vi "FTW-Actor-LaunchChildActor-Path.vi"(0 "FTW-ActorInstance In":refnum<class "FTW-ActorInstance.lvclass">, 5 "Configuration":string="{\n  \"Identity\": \"ActorName\",\n  \"DebugEnableInboxLogging\": false,\n  \"DebugEnableJobLogging\": false,\n  \"InboxAddress\": \"inproc://*\",\n  \"DebugShowPanel\": false\n}", 7 "Actor VI Path":path, 9 "Timeout":i32=-2 format="%dmsec", 11 "error in":errorcluster) -> (4 "FTW-ActorInstance Out":refnum<class "FTW-ActorInstance.lvclass">, 6 "Initialized Response":string, 8 "Instance Inbox Address":string, 10 "Identity":string, 15 "error out":errorcluster)   [LabVIEW 2018, in "FTW-ActorInstance.lvclass"]
doc: "This is the spawn new actor that was used for a while. It lacks the minimum strict inputs required to launch an actor."
uses:
  FTW-ActorInstance.lvclass
  Connector/FTW-ActorConnector.lvclass
  4a73fd1e-9fc2-4821-946b-9eb06f56bf7f.vi
  JSON/core/FTW-JSON-Core-EncodingFlags.vi
  Reflection/FTW-Reflection-Type.vi
  JSON/FTW-JSON-Parse.vi
  container/FTW-Container-GetFlattenedValue.vi
panel:
  # "Inputs"
  # "Outputs"
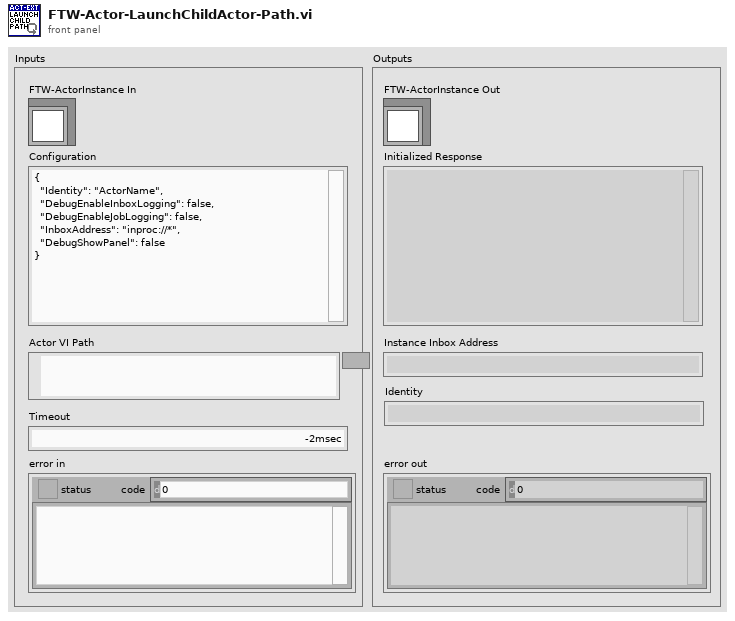
[diagram p1: front panel]
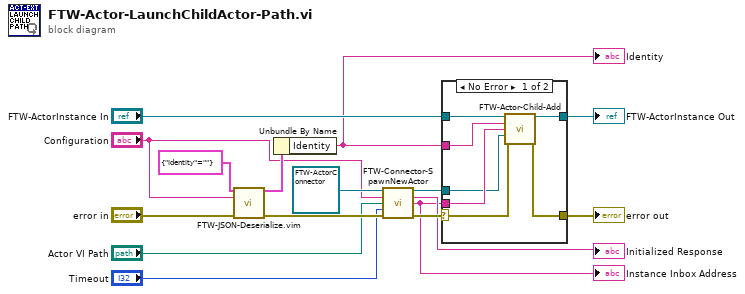
[diagram p0: block diagram]
diagram:
  n1 = call "FTW-JSON-Deserialize.vim"("Type In"=cluster{"Identity":string} {"Identity"=""}, "JSON String"="Configuration", "error in"="error in") -> ("Type Out"=w15:cluster{"Identity":string}, "error out"=w13:errorcluster)  [unwired: 11 in]
  n2 = Unbundle By Name(w15) -> ("Identity"=w2:string)
  "Identity" <- w2
  n3 = call "FTW-Connector-SpawnNewActor.vi"("FTW Actor Connector Type"=refnum<class "FTW-ActorConnector.lvclass"> refnum, "Configuration"="Configuration", "Actor VI Filepath"="Actor VI Path", "Timeout"="Timeout", "error in"=w13) -> ("FTW Actor Connector"=w11:refnum<class "FTW-ActorConnector.lvclass">, "Initialized Response"=→"Initialized Response":string, "Instance Inbox Address"=w5:string, "error out"=w12:errorcluster)  [unwired: 7 in]
  "Instance Inbox Address" <- w5
  n4 = case shown="No Error" w12 {
    selector: w12 -> [w23 w24]
    tunnel: "FTW-ActorInstance In" -> [w21 w25]
    tunnel: [w20 w25] -> w7
    tunnel: [w22 w24] -> w4
    tunnel: w2 -> [w19 _]
    tunnel: w5 -> [w18 _]
    tunnel: w11 -> [w17 _]
    frame No Error {
      n5 = call "FTW-Actor-Child-Add.vi"("FTW-ActorExtended In"=w21, "Identity"=w19, "Inbox Address"=w18, "Connection"=w17, "error in"=w23) -> ("FTW-ActorExtended Out"=w20:refnum<class "FTW-ActorInstance.lvclass">, "error out"=w22:errorcluster)  [unwired: 9 in]
    }
    frame Error {
    }
  }
  "error out" <- w4
  "FTW-ActorInstance Out" <- w7
